vi "Find All Folders in Project.vi"(5 "Exclude Own Project Files?(T)":bool=TRUE, 7 "To Lower Case?(T)":bool=TRUE, 8 "error in (no error)":errorcluster, 11 "Project Path":path) -> (0 "error out":errorcluster, 1 "Success?":bool, 3 "Project Folders":string[](array[string]))   [LabVIEW 2019, in "Project.Dependencies Finder.lvlib"]
doc: "Extract all files from project at 'Project Path'."
uses:
  Project.Dependencies Finder.lvlib
  247e5f67-52b4-4194-899c-141e10737219.vi
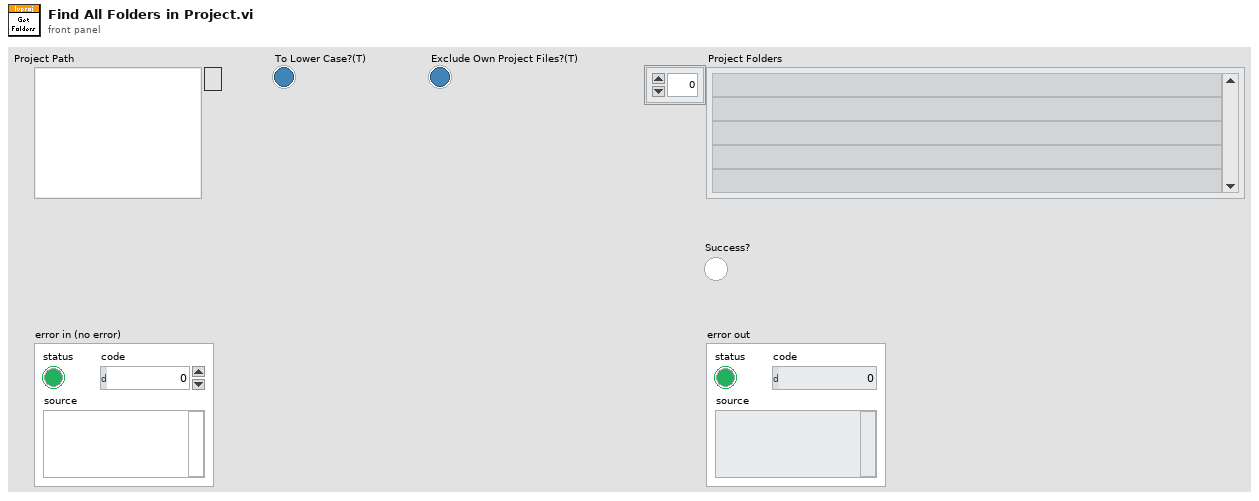
[diagram p1: front panel]
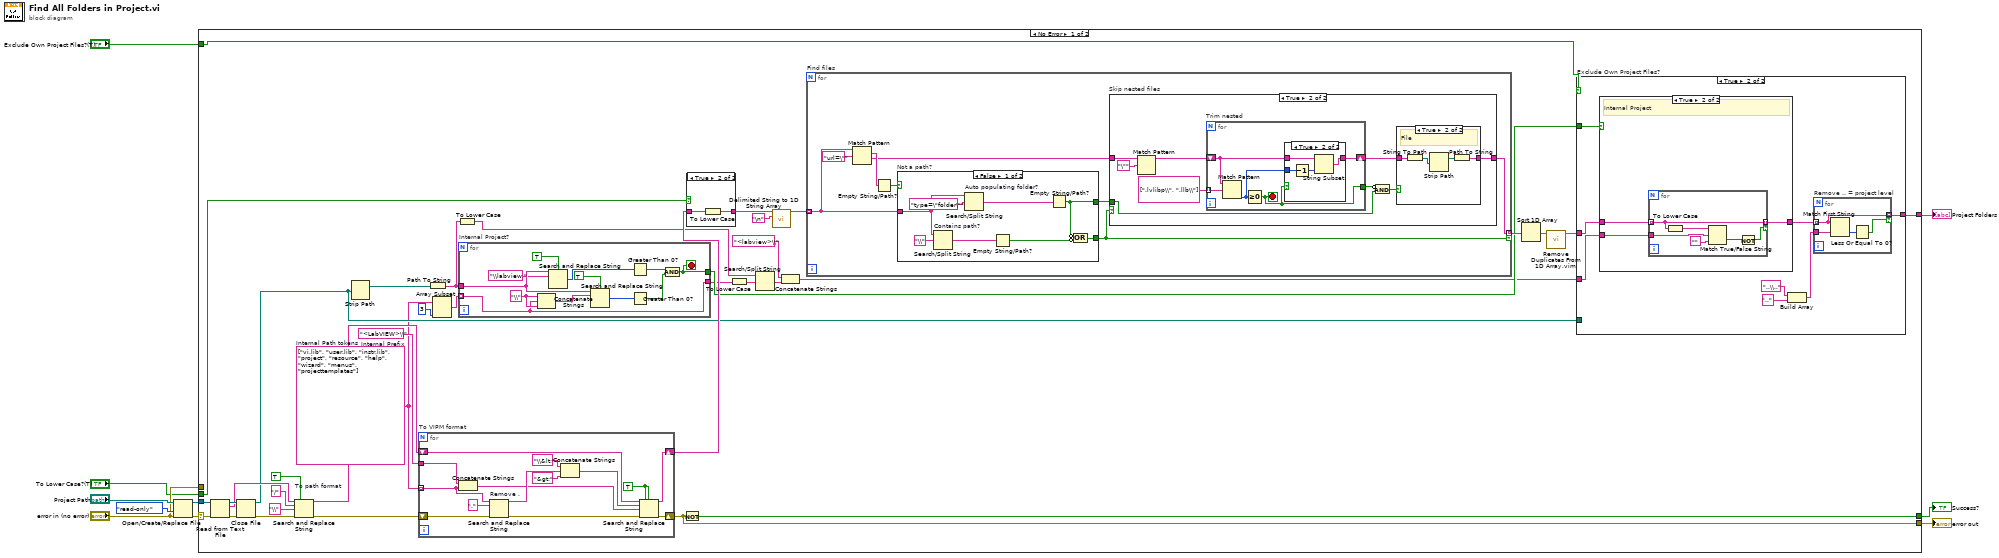
[diagram p0: block diagram]
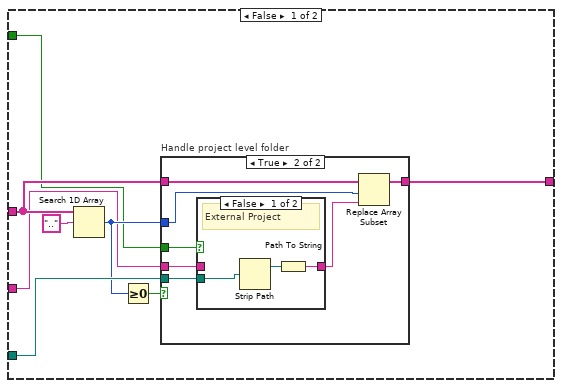
[diagram p2: hidden frame]
diagram:
  n1 = Open/Create/Replace File(file path (use dialog)="Project Path", error in="error in (no error)", access (0:read/write)=enum16{"read/write", "read-only", "write-only"}."read-only") -> (refnum out=w6:refnum<file>, error out=w7:errorcluster)  [unwired: 3 in, 1 out]
  n2 = case shown="No Error" w7 {
    selector: w7 -> [w33 _]
    tunnel: [w26 _] -> w10
    tunnel: [w30 w159] -> w8
    tunnel: w6 -> [w32 _]
    tunnel: "error in (no error)" -> [_ w159]
    tunnel: [w29 _] -> w3
    tunnel: "To Lower Case?(T)" -> [w28 _]
    tunnel: "Exclude Own Project Files?(T)" -> [w27 _]
    frame No Error {
      w46 = "<LabVIEW>\\"  # Internal Prefix
      w23 = string[] ["vi.lib", "user.lib", "instr.lib", "project", "resource", "help", "wizard", "menus", "projecttemplates"]  # Internal Path tokens
      n3 = Read from Text File(file (use dialog)=w32, error in=w33) -> (refnum out=w34:refnum<file>, text=w31:string, error out=w35:errorcluster)  [unwired: 2 in, 1 out]
      n4 = Close File(refnum=w34, error in=w35) -> (path=w24:path, error out=w44:errorcluster)
      n5 = Search and Replace String "To path format"(replace all?=TRUE ("replace all? (F)"), input string=w31, search string="/" ("String"), replace string="\\" ("replace string (\"\")"), error in=w44) -> (result string=w40:string, error out=w45:errorcluster)  [unwired: 3 in, 2 out]
      n6 = Strip Path(path=w24) -> (stripped path=w21:path)  [unwired: 1 out]
      n7 = for "To VIPM format" {
        shift-right: [w117] -> w36
        shift-left: w40 -> [w118]
        shift-right: [w116] -> w30
        shift-left: w45 -> [w107]
        tunnel: w23 -> [w109] mode=indexing
        tunnel: w46 -> [w105]
        w115 = TRUE ("replace all? (F)")
        n8 = Concatenate Strings(w105, w109) -> (w108:string)
        n9 = Search and Replace String "Remove ."(input string=w109, search string="." ("String"), error in=w107) -> (result string=w113:string, error out=w106:errorcluster)  [unwired: 5 in, 2 out]
        n10 = Concatenate Strings("\\&lt;", w113, "&gt;" ("string")) -> (w110:string)
        n11 = Search and Replace String(replace all?=w115, case sensitive?=w115, input string=w118, search string=w110, replace string=w108, error in=w106) -> (result string=w117:string, error out=w116:errorcluster)  [unwired: 2 in, 2 out]
      }
      n12 = Path To String(path=w21) -> (string=w13:string)
      n13 = Array Subset(array=w23, length=3) -> (w20:string[])  [unwired: 1 in]
      n14 = To Lower Case(string=w13) -> (all lower case string=w16:string)
      n15 = for "Internal Project?" {
        tunnel: w13 -> [w53]
        tunnel: w20 -> [w54] mode=indexing
        tunnel: [w50] -> w18
        tunnel: [w54] -> w12
        stop <- w50 stop-if-true
        w59 = "\\" ("string")
        n16 = Concatenate Strings(w59, w54, w59) -> (w57:string)
        n17 = Search and Replace String(case sensitive?=TRUE ("replace all? (F)"), input string=w53, search string="\\labview ") -> (number of replacements=w51:i32)  [unwired: 5 in, 3 out]
        n18 = Search and Replace String(case sensitive?=TRUE ("replace all? (F)"), input string=w53, search string=w57) -> (number of replacements=w56:i32)  [unwired: 5 in, 3 out]
        n19 = Greater Than 0?(x=w51) -> (x > 0?=w49:bool)
        n20 = Greater Than 0?(x=w56) -> (x > 0?=w55:bool)
        n21 = And(x=w49, y=w55) -> (x .and. y?=w50:bool)
      }
      n22 = Not(x=w30) -> (.not. x?=w29:bool)
      n23 = case shown="True" w28 {
        tunnel: [w102 w104] -> w37
        tunnel: w36 -> [w102 w103]
        frame False {
        }
        frame True {
          n24 = To Lower Case(string=w103) -> (all lower case string=w104:string)
        }
      }
      n25 = To Lower Case(string=w12) -> (all lower case string=w17:string)
      n26 = Search/Split String(string=w16, search string/char (-)=w17) -> (match + rest of string=w15:string)  [unwired: 1 in, 2 out]
      n27 = call <vilib>:"Delimited String to 1D String Array.vi"("delimiter"="\n", "delimited string"=w37) -> ("string array"=w47:string[])  [unwired: 9 in]
      n28 = Concatenate Strings("<labview>\\" ("string"), w15) -> (w11:string)
      n29 = for "Find files" {
        tunnel: w47 -> [w123] mode=indexing
        tunnel: [w124] -> w39 mode=indexing if=w121
        n30 = Match Pattern(string=w123, regular expression="url=\"") -> (match substring=w125:string, after substring=w122:string)  [unwired: 1 in, 2 out]
        n31 = Empty String/Path?(string/path=w125) -> (empty?=w120:bool)
        n32 = case "Not a path?" shown="False" w120 {
          tunnel: w123 -> [w131 _]
          tunnel: [w128 _] -> w121
          tunnel: [w127 _] -> w119
          frame False {
            n33 = Search/Split String "Contains path?"(string=w131, search string/char (-)="\\") -> (match + rest of string=w133:string)  [unwired: 1 in, 2 out]
            n34 = Search/Split String "Auto populating folder?"(string=w131, search string/char (-)="type=\"folder\"") -> (match + rest of string=w129:string)  [unwired: 1 in, 2 out]
            n35 = Empty String/Path?(string/path=w133) -> (empty?=w132:bool)
            n36 = Empty String/Path?(string/path=w129) -> (empty?=w127:bool)
            n37 = Compound Arithmetic op=OR(invert w127, invert w132) -> (w128:bool)
          }
          frame True {
          }
        }
        n38 = case "Skip nested files" shown="True" w121 {
          tunnel: [_ w135] -> w124
          tunnel: w122 -> [_ w142]
          tunnel: w119 -> [_ w139]
          frame False {
          }
          frame True {
            n39 = Match Pattern(string=w142, regular expression="\"") -> (before substring=w140:string)  [unwired: 1 in, 3 out]
            n40 = for "Trim nested" {
              tunnel: string[] [".lvlibp\\", ".llb\\"] ("regular expression") -> [w153] mode=indexing
              shift-right: [w150] -> w136
              shift-left: w140 -> [w152]
              tunnel: [w149] -> w138
              stop <- w149 stop-if-true
              n41 = Match Pattern(string=w152, regular expression=w153) -> (offset past match=w151:i32)  [unwired: 1 in, 3 out]
              n42 = Greater Or Equal To 0?(x=w151) -> (x >= 0?=w149:bool)
              n43 = case shown="True" w149 {
                tunnel: w152 -> [w154 w158]
                tunnel: w151 -> [_ w157]
                tunnel: [w154 w156] -> w150
                frame False {
                }
                frame True {
                  n44 = Decrement(x=w157) -> (x-1=w155:i32)
                  n45 = String Subset(string=w158, length (rest)=w155) -> (substring=w156:string)  [unwired: 1 in]
                }
              }
            }
            n46 = Compound Arithmetic op=AND(invert w138, w139) -> (w137:bool)
            n47 = case shown="True" w137 {
              tunnel: [w144 w145] -> w135
              tunnel: w136 -> [w144 w148]
              frame False {
                # "Folder"
              }
              frame True {
                # "File"
                n48 = String To Path(string=w148) -> (path=w147:path)
                n49 = Strip Path(path=w147) -> (stripped path=w146:path)  [unwired: 1 out]
                n50 = Path To String(path=w146) -> (string=w145:string)
              }
            }
          }
        }
      }
      n51 = Sort 1D Array(array=w39) -> (sorted array=w25:string[])
      n52 = call "Remove Duplicates From 1D Array.vim"("array"=w25) -> ("array with duplicates removed"=w22:string[])  [unwired: 10 in]
      n53 = case "Exclude Own Project Files?" shown="True" w27 {
        tunnel: [w64 w82] -> w26
        tunnel: w22 -> [w65 w87]
        tunnel: w24 -> [w63 _]
        tunnel: w18 -> [w61 w81]
        tunnel: w11 -> [w60 w80]
        frame False {
          n54 = Search 1D Array(1D array=w65, element="..") -> (index of element=w62:i32)  [unwired: 1 in]
          n55 = Greater Or Equal To 0?(x=w62) -> (x >= 0?=w66:bool)
          n56 = case "Handle project level folder" shown="True" w66 {
            tunnel: [w68 w71] -> w64
            tunnel: w65 -> [w68 w74]
            tunnel: w63 -> [_ w75]
            tunnel: w62 -> [_ w73]
            tunnel: w61 -> [_ w70]
            tunnel: w60 -> [_ w69]
            frame False {
            }
            frame True {
              n57 = case shown="False" w70 {
                tunnel: w75 -> [w78 _]
                tunnel: [w76 w79] -> w72
                tunnel: w69 -> [_ w79]
                frame False {
                  # "External Project"
                  n58 = Strip Path(path=w78) -> (stripped path=w77:path)  [unwired: 1 out]
                  n59 = Path To String(path=w77) -> (string=w76:string)
                }
                frame True {
                  # "Internal Project"
                }
              }
              n60 = Replace Array Subset(array=w74, new element=w72, index=w73) -> (w71:string[])
            }
          }
        }
        frame True {
          n61 = case shown="True" w81 {
            tunnel: w87 -> [w92 w95]
            tunnel: [w92 w94] -> w83
            tunnel: w80 -> [_ w93]
            frame False {
              # "External Project"
            }
            frame True {
              # "Internal Project"
              n62 = for {
                tunnel: w93 -> [w98]
                tunnel: w95 -> [w101] mode=indexing
                tunnel: [w101] -> w94 mode=indexing if=w96
                n63 = To Lower Case(string=w101) -> (all lower case string=w99:string)
                n64 = Match True/False String(2:"" ("true string"), 3:w98, 4:w99) -> (0:w100:bool)  [unwired: 1 out]
                n65 = Not(x=w100) -> (.not. x?=w96:bool)
              }
            }
          }
          n66 = Build Array("..\\..", "..") -> (w86:string[])
          n67 = for "Remove .. = project level" {
            tunnel: w83 -> [w89] mode=indexing
            tunnel: w86 -> [w91]
            tunnel: [w89] -> w82 mode=indexing if=w88
            n68 = Match First String(2:w91, 3:w89) -> (0:w90:i32)  [unwired: 1 out]
            n69 = Less Or Equal To 0?(x=w90) -> (x <= 0?=w88:bool)
          }
        }
      }
    }
    frame Error {
    }
  }
  "Project Folders" <- w10
  "error out" <- w8
  "Success?" <- w3
